vi "Test GitHub Issue 30 - Deserialize Array of Cluster of Multi-Dimensional Array Wraps Inner Elements in Variants.vi"(8 "error in (no error)":errorcluster) -> (0 "error out":errorcluster)   [LabVIEW 2013]
uses:
  src/Serializer/JSON Serializer/JSON Serializer.lvclass
  src/Deserializer/JSON Deserializer/JSON Deserializer.lvclass
  <vilib>/addons/_JKI Toolkits/Caraya/classes/Test/Test.lvclass
  <vilib>/addons/_JKI Toolkits/Caraya/classes/Assert/Assert.lvclass
panel:
  out "Pass?":bool
  out "JSON":string
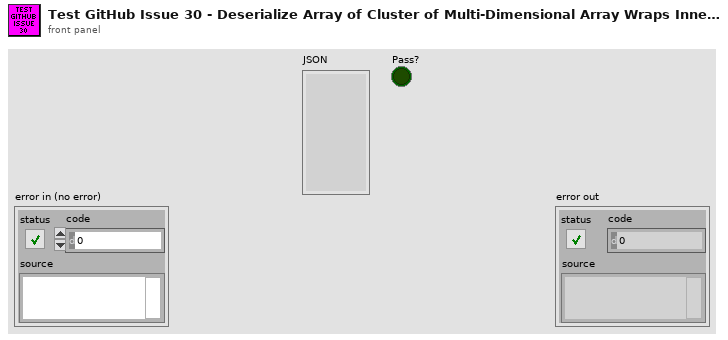
[diagram p1: front panel]
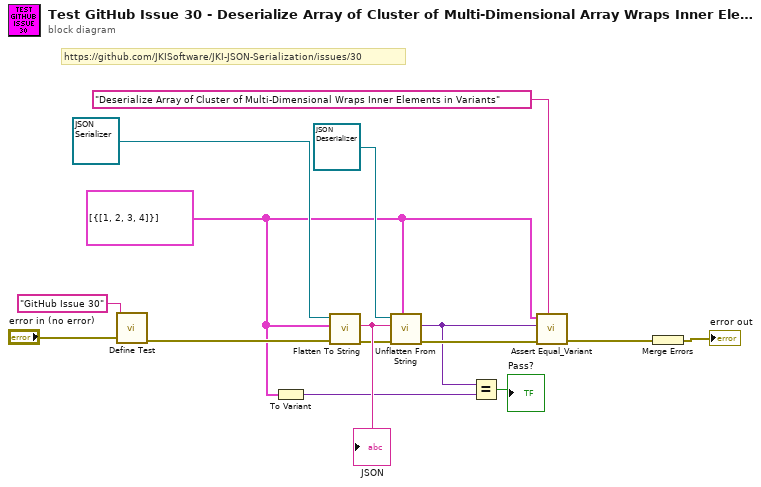
[diagram p0: block diagram]
diagram:
  w5 = cluster{i32[][]}[] [{[[1, 2], [3, 4]]}]
  # "https://github.com/JKISoftware/JKI-JSON-Serialization/issues/30"
  n1 = call <vilib>:"Define Test.vi"("error in (no error)"="error in (no error)", "Label (VI Title)"="GitHub Issue 30") -> ("error out"=w13:errorcluster)  [unwired: 9 in]
  n2 = To Variant(anything=w5) -> (Variant=w1:variant)
  n3 = call-dynamic "Flatten To String.vi"("error in (no error)"=w13, "Variant"=w5, "JSON Serializer in"=refnum<class "JSON Serializer.lvclass"> refnum ("JKI JSON Serialization.lvlib:JSON Serializer.lvclass")) -> ("error out"=w8:errorcluster, "String"=w9:string)  [unwired: 6 in, 1 out]
  "JSON" <- w9
  n4 = call-dynamic "Unflatten From String.vi"("Type and Defaults"=w5, "error in (no error)"=w8, "String"=w9, "Deserializer in"=refnum<class "JSON Deserializer.lvclass"> refnum) -> ("error out"=w7:errorcluster, "Variant"=w2:variant)  [unwired: 5 in, 1 out]
  n5 = Equal?(x=w2, y=w1) -> (x = y?=→"Pass?":bool)
  n6 = call <vilib>:"Assert Equal_Variant.vi"("Label"="Deserialize Array of Cluster of Multi-Dimensional Wraps Inner Elements in Variants", "error in (no error)"=w7, "Y"=w2, "X"=w5) -> ("error out"=w12:errorcluster)  [unwired: 7 in]
  n7 = Merge Errors(w12) -> (→"error out":errorcluster)
